vi "Calibrate Pneumotach.vi"(11 "Error In":errorcluster) -> (15 "Error Out":errorcluster)   [LabVIEW 2020]
uses:
  <vilib>/Analysis/baseanly.llb/Mean (DBL).vi
  <vilib>/measure/madcrms.llb/Basic Averaged DC-RMS for 1 Chan.vi
  <vilib>/gmath/NI_Gmath.lvlib
  <vilib>/Analysis/NI_AALBase.lvlib
  <vilib>/measure/NI_MAPro.lvlib
panel:
  in  "Remove Button":bool
  out "Flow Array":dbl[](array[numeric]) format="%_6g"
  out "Flow Calibration":cluster{"Y":dbl[], "Y":dbl[]}[](graph)
  out "Pressure Slope":dbl
  out "Pressure Intercept":dbl
  out "Pressure Voltage":dbl
  out "Flow Voltage":dbl
  in  "Flow Reference":dbl min=0.0 max=30.0 step=6.0
  out "Flow Intercept":dbl
  out "Flow Slope":dbl
  in  "Stop Button HS":bool
  in  "Add Button HS":bool
  out "Flow Curve":cluster{"Y":dbl[], "Y":dbl[]}[](graph)
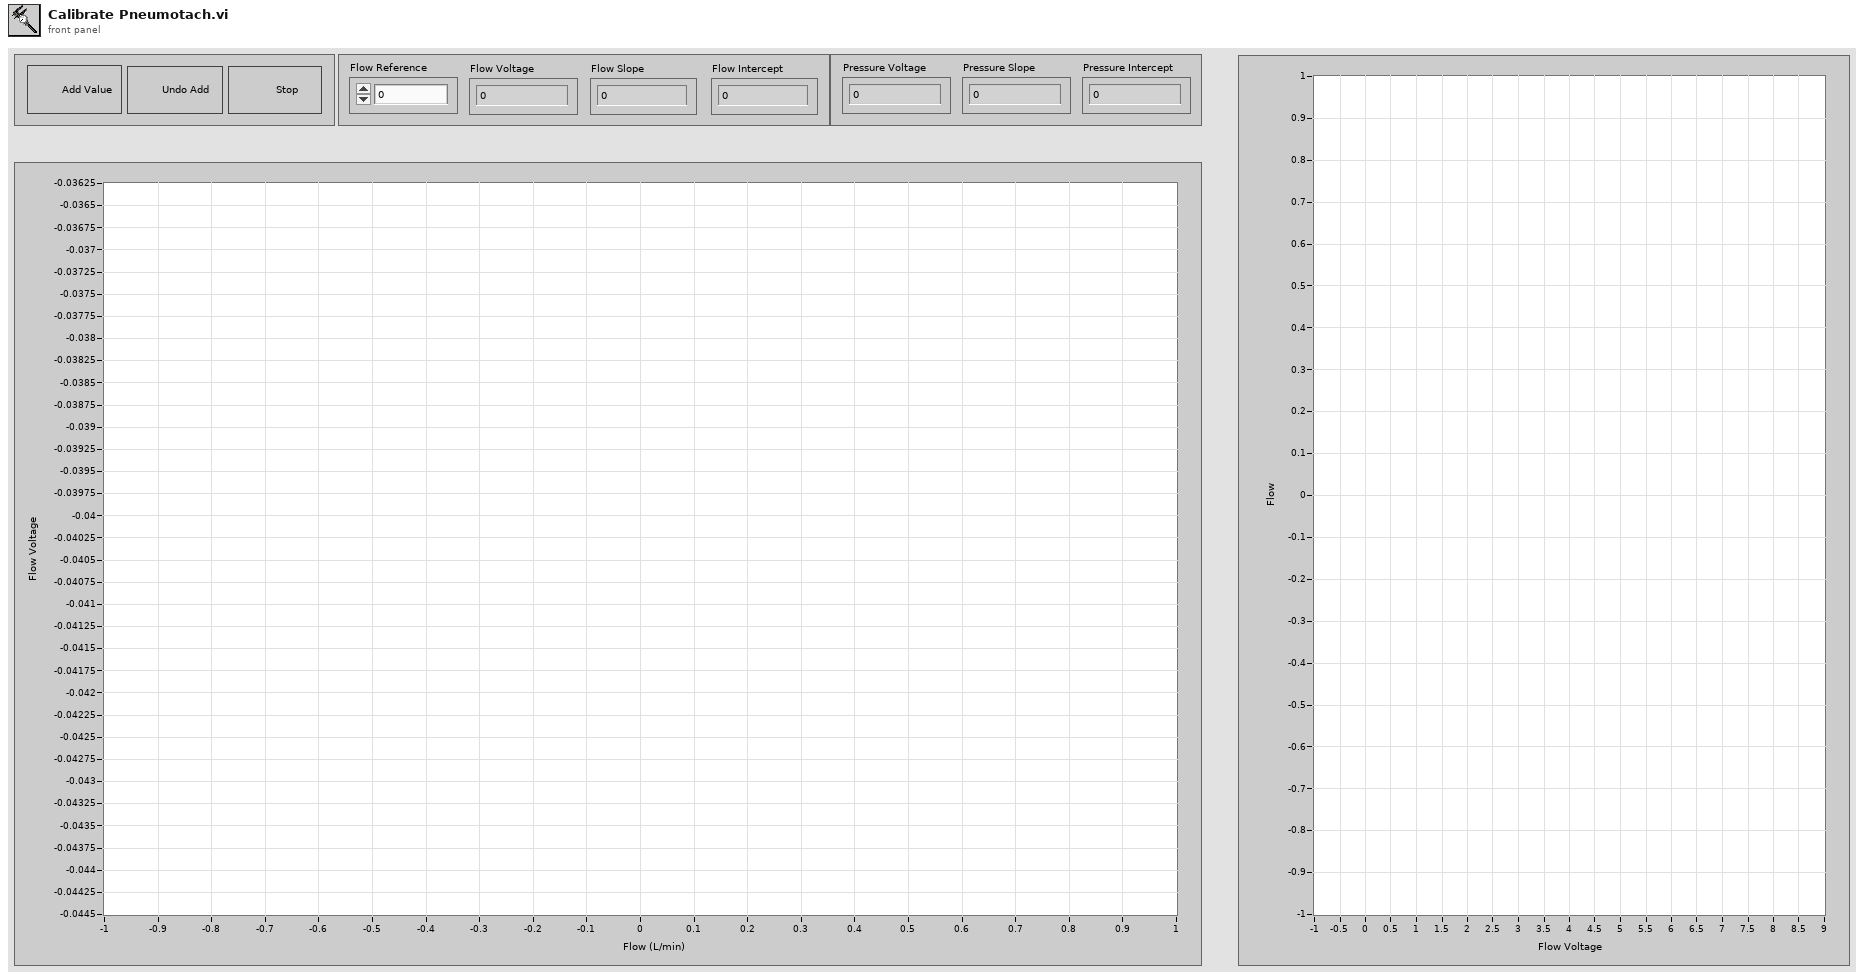
[diagram p1: front panel]
types:
  T1 = enum16{"open", "replace", "create", "open or create", "replace or create", "replace or create with confirmation"}
  T2 = enum8{"Enabled", "Disabled", "Disabled and Grayed Out"}
  T3 = cluster{"Volt (Flow)":dbl[], "Ref (Flow)":dbl[]}[]
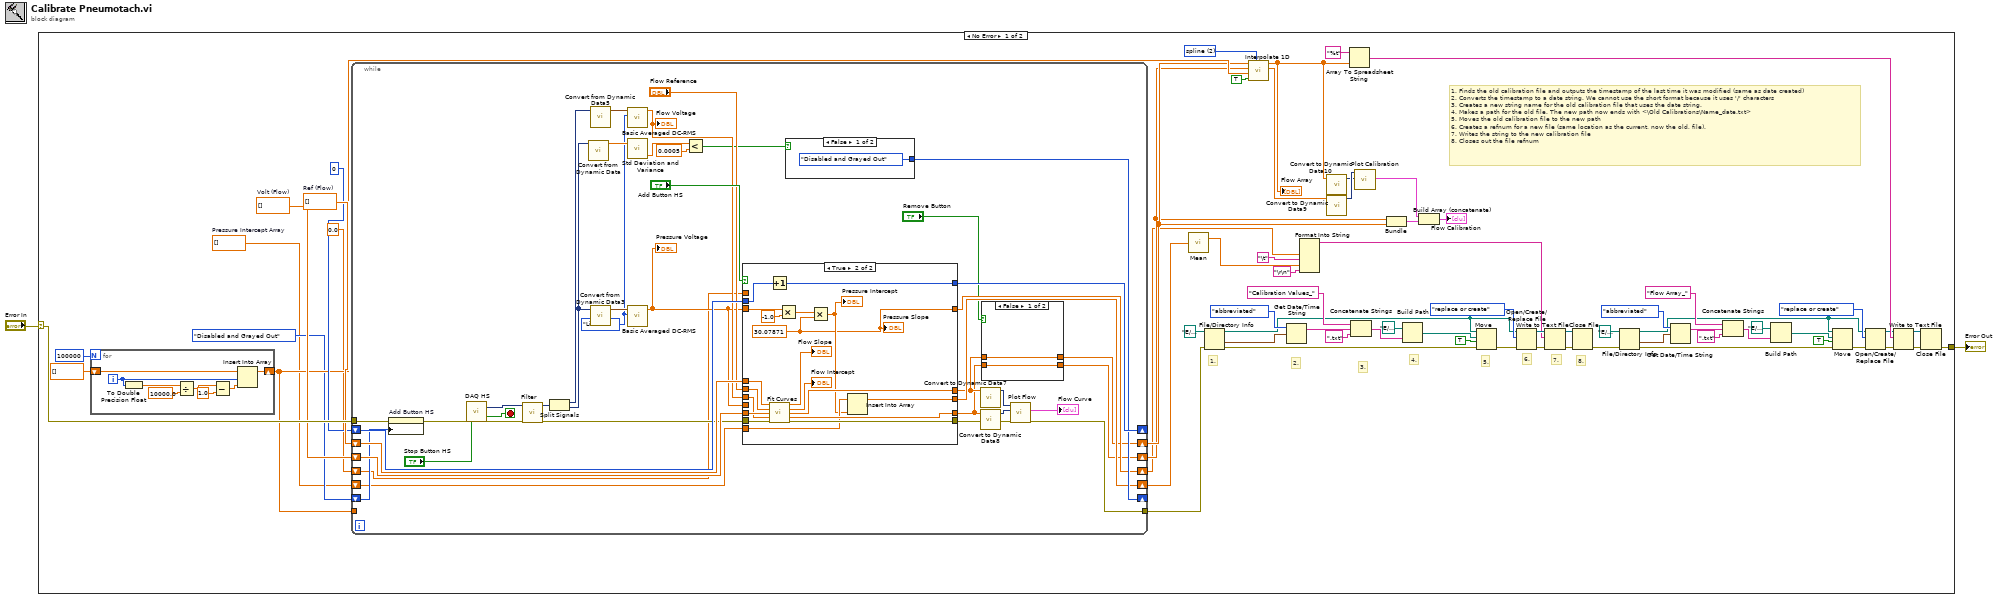
[diagram p0: block diagram]
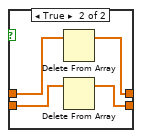
[diagram p2: hidden frame]
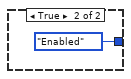
[diagram p3: hidden frame]
diagram:
  n1 = case shown="No Error" "Error In" {
    selector: "Error In" -> [w70 w153]
    tunnel: [w43 w153] -> w1
    frame No Error {
      w24 = dbl[] []  # Pressure Intercept Array
      w65 = 2 items=["nearest", "linear", "spline", "cubic Hermite", "Lagrange"] ("method")
      w68 = dbl[] []  # Ref (Flow)
      w69 = dbl[] []  # Volt (Flow)
      # "1. Finds the old calibration file and outputs the timestamp of the last time it was modified (same as date created)\n2. Converts the timestamp to a date string. We cannot use the short format because it uses '/' characters\n3. Creates a new string name for the old calibration file that uses the date string.\n4. Makes a path for the old file. The new path now ends with <\\Old Calibrations\\Name_date.txt>\n5. Moves the old calibration file to the new path\n6. Creates a refnum for a new file (same location as the current, now the old, file).\n7. Writes the string to the new calibration file\n8. Closes out the file refnum"
      # "8."
      # "7."
      # "6."
      # "5."
      # "4."
      # "3."
      # "2."
      # "1."
      n2 = for {
        N: 100000 ("dimension size") -> [_]
        shift-right: [w77] -> w59
        shift-left: dbl[] [] -> [w78]
        i -> [w74]
        n3 = To Double Precision Float(number=w74) -> (double precision float=w75:dbl)
        n4 = Divide(x=w75, y=10000.0) -> (x/y=w73:dbl)
        n5 = Subtract(x=w73, y=1.0) -> (x-y=w71:dbl)
        n6 = Insert Into Array(array=w78, index=w74, new element=w71) -> (w77:dbl[])
      }
      n7 = while {
        tunnel: w70 -> [w103]
        shift-right: [w79] -> w54
        shift-left: w69 -> [w106]
        shift-right: [w81] -> w55
        shift-left: w68 -> [w108]
        tunnel: [w111] -> w33
        shift-right: [w109] -> _
        shift-left: 0 -> [w110]
        tunnel: w59 -> [_]
        shift-right: [w100] -> _
        shift-left: T2."Disabled and Grayed Out" ("Disabled") -> [w101]
        shift-right: [w86] -> w23
        shift-left: w24 -> [w87]
        shift-right: [w84] -> w4
        shift-left: 0.0 -> [w85]
        stop <- w115 stop-if-true
        w92 = enum16{"Linear", "Exponential"}."Linear" ("averaging type")
        n8 = property on="Add Button HS" class="Bool"(error in=w103, "DisabledEnum"=w101) -> (error out=w102:errorcluster)  [unwired: 1 in, 1 out]
        n9 = call "DAQ HS"("error in"=w102, "stop (F)"="Stop Button HS") -> ("data"=w118:dynamicdata, "stopped"=w115:bool, "error out"=w119:errorcluster)  [unwired: 14 in, 1 out]
        n10 = call "Filter"("error in (no error)"=w119, "Signal"=w118) -> ("error out"=w93:errorcluster, "Filtered Signal"=w104:dynamicdata)  [unwired: 8 in]
        n11 = Split Signals(w104) -> (w89:dynamicdata, w95:dynamicdata)  [unwired: 2 in]
        n12 = call "Convert from Dynamic Data"("Dynamic Data Type"=w95) -> ("Array"=w98:dbl[])  [unwired: 3 in]
        n13 = call "Convert from Dynamic Data5"("Dynamic Data Type"=w89) -> ("Waveform"=w94:waveform(dbl))  [unwired: 3 in]
        n14 = call "Convert from Dynamic Data3"("Dynamic Data Type"=w95) -> ("Waveform"=w96:waveform(dbl))  [unwired: 3 in]
        n15 = call-poly <vilib>:"Basic Averaged DC-RMS.vi"("averaging type"=w92, "signal in"=w94) -> ("DC value"=w91:dbl)  [unwired: 6 in, 3 out]
        "Flow Voltage" <- w91
        n16 = call <vilib>:"Std Deviation and Variance.vi"("X"=w98) -> ("variance"=w97:dbl)  [unwired: 1 in, 2 out]
        n17 = call-poly <vilib>:"Basic Averaged DC-RMS.vi"("averaging type"=w92, "signal in"=w96) -> ("DC value"=w88:dbl)  [unwired: 6 in, 3 out]
        "Pressure Voltage" <- w88
        n18 = Less?(x=w97, y=0.0005) -> (x < y?=w90:bool)
        n19 = case shown="True" "Add Button HS" {
          tunnel: w93 -> [w133 w149]
          tunnel: [w133 w150] -> w114
          tunnel: w110 -> [w132 w152]
          tunnel: [w132 w151] -> w109
          tunnel: w108 -> [w131 w148]
          tunnel: "Flow Reference" -> [_ w147]
          tunnel: w106 -> [w130 w146]
          tunnel: w91 -> [_ w145]
          tunnel: [w131 w142] -> w82
          tunnel: [w130 w141] -> w80
          tunnel: w88 -> [_ _]
          tunnel: w88 -> [_ w136]
          tunnel: [w128 w134] -> w84
          tunnel: w87 -> [w129 w140]
          tunnel: [w129 w139] -> w86
          tunnel: w85 -> [w128 _]
          frame False {
          }
          frame True {
            w134 = 30.07871
            n20 = Increment(x=w152) -> (x+1=w151:i32)
            n21 = call "Fit Curves.vi"("Reference (Array)"=w148, "Reference (Value)"=w147, "Voltage (Array)"=w146, "Voltage (Value)"=w145, "Error In"=w149) -> ("Slope"=→"Flow Slope":dbl, "Intercept"=→"Flow Intercept":dbl, "Reference Out"=w142:dbl[], "Voltage Out"=w141:dbl[], "Error Out"=w150:errorcluster)  [unwired: 6 in]
            n22 = Multiply(x=w136, y=-1.0) -> (x*y=w135:dbl)
            n23 = Multiply(x=w135, y=w134) -> (x*y=w137:dbl)
            "Pressure Intercept" <- w137
            n24 = Insert Into Array(array=w140, new element=w137) -> (w139:dbl[])  [unwired: 1 in]
            "Pressure Slope" <- w134
          }
        }
        n25 = case shown="False" w90 {
          tunnel: [T2."Disabled and Grayed Out" ("Disabled") T2."Enabled" ("Disabled")] -> w100
          frame False {
          }
          frame True {
          }
        }
        n26 = call "Convert to Dynamic Data7"("Array"=w82) -> ("Dynamic Data Type"=w112:dynamicdata)  [unwired: 3 in]
        n27 = call "Convert to Dynamic Data8"("Array"=w80) -> ("Dynamic Data Type"=w113:dynamicdata)  [unwired: 3 in]
        n28 = case shown="False" "Remove Button" {
          tunnel: w82 -> [w121 w125]
          tunnel: [w121 w124] -> w81
          tunnel: w80 -> [w120 w123]
          tunnel: [w120 w122] -> w79
          frame False {
          }
          frame True {
            n29 = Delete From Array(array=w125) -> (array with subset deleted=w124:dbl[])  [unwired: 2 in, 1 out]
            n30 = Delete From Array(array=w123) -> (array with subset deleted=w122:dbl[])  [unwired: 2 in, 1 out]
          }
        }
        n31 = call "Plot Flow"("error in (no error)"=w114, "Y Input"=w113, "X Input"=w112) -> ("error out"=w111:errorcluster, "XY Graph"=→"Flow Curve":cluster{"Y":dbl[], "Y":dbl[]}[])  [unwired: 7 in]
      }
      n32 = call-poly <vilib>:"Mean.vi"("X"=w23) -> ("mean"=w3:dbl)  [unwired: 1 out]
      n33 = File/Directory Info(path=path "E:/Program Files/Master Aero Program/Calibration .txt files/Calibration Values.txt" ("file path (use dialog)"), error in=w33) -> (path out=w26:path, last mod=w30:timestamp, error out=w34:errorcluster)  [unwired: 4 out]
      n34 = call <vilib>:"Interpolate 1D.vi"("method"=w65, "X is monotonic"=TRUE, "xi"=w59, "X"=w54, "Y"=w55) -> ("xi used"=w57:dbl[], "yi"=w46:dbl[])  [unwired: 4 in, 1 out]
      "Flow Array" <- w46
      n35 = Get Date/Time String(date format (0)=enum16{"short", "long", "abbreviated"}."abbreviated", seconds (now)=w30) -> (date string=w29:string)  [unwired: 1 in, 1 out]
      n36 = Format Into String(w4, "\t", w3, "\r\n") -> (resulting string=w49:string)  [unwired: 3 in, 1 out]
      n37 = call "Convert to Dynamic Data10"("Array"=w46) -> ("Dynamic Data Type"=w63:dynamicdata)  [unwired: 3 in]
      n38 = call "Convert to Dynamic Data9"("Array"=w57) -> ("Dynamic Data Type"=w64:dynamicdata)  [unwired: 3 in]
      n39 = Array To Spreadsheet String(array=w46, 3:"%t" ("format string")) -> (spreadsheet string=w41:string)  [unwired: 1 in]
      n40 = Concatenate Strings("Calibration Values_" ("string"), w29, ".txt" ("string")) -> (w36:string)
      n41 = call "Plot Calibration"("Y Input"=w63, "X Input"=w64) -> ("XY Graph"=w62:cluster{"Y":dbl[], "Y":dbl[]}[])  [unwired: 8 in, 1 out]
      n42 = Bundle("Volt (Flow)"=w54, "Ref (Flow)"=w55) -> (w61:cluster{"Volt (Flow)":dbl[], "Ref (Flow)":dbl[]})  [unwired: 1 in]
      n43 = Build Path(base path=path "E:/Program Files/Master Aero Program/Calibration .txt files/Old Calibrations" ("target path (use dialog)"), name or relative path=w36) -> (appended path=w39:path)
      n44 = Build Array (concatenate)(w62, w61) -> (→"Flow Calibration":T3)
      n45 = Move(source path=w26, error in=w34, 9:TRUE ("overwrite (F)"), 10:w39) -> (error out=w40:errorcluster)  [unwired: 1 in, 2 out]
      n46 = Open/Create/Replace File(file path (use dialog)=w26, error in=w40, operation (0:open)=T1."replace or create") -> (refnum out=w51:refnum<file>, error out=w35:errorcluster)  [unwired: 3 in, 1 out]
      n47 = Write to Text File(file (use dialog)=w51, text=w49, error in=w35) -> (refnum out=w50:refnum<file>, error out=w52:errorcluster)  [unwired: 1 in, 1 out]
      n48 = Close File(refnum=w50, error in=w52) -> (error out=w28:errorcluster)  [unwired: 1 out]
      n49 = File/Directory Info(path=path "E:/Program Files/Master Aero Program/Calibration .txt files/Flow Array.txt" ("file path (use dialog)"), error in=w28) -> (path out=w6:path, last mod=w8:timestamp, error out=w15:errorcluster)  [unwired: 4 out]
      n50 = Get Date/Time String(date format (0)=enum16{"short", "long", "abbreviated"}."abbreviated", seconds (now)=w8) -> (date string=w7:string)  [unwired: 1 in, 1 out]
      n51 = Concatenate Strings("Flow Array_" ("string"), w7, ".txt" ("string")) -> (w12:string)
      n52 = Build Path(base path=path "E:/Program Files/Master Aero Program/Calibration .txt files/Old Calibrations" ("target path (use dialog)"), name or relative path=w12) -> (appended path=w16:path)
      n53 = Move(source path=w6, error in=w15, 9:TRUE ("overwrite (F)"), 10:w16) -> (error out=w17:errorcluster)  [unwired: 1 in, 2 out]
      n54 = Open/Create/Replace File(file path (use dialog)=w6, error in=w17, operation (0:open)=T1."replace or create") -> (refnum out=w20:refnum<file>, error out=w19:errorcluster)  [unwired: 3 in, 1 out]
      n55 = Write to Text File(file (use dialog)=w20, text=w41, error in=w19) -> (refnum out=w21:refnum<file>, error out=w18:errorcluster)  [unwired: 1 in, 1 out]
      n56 = Close File(refnum=w21, error in=w18) -> (error out=w43:errorcluster)  [unwired: 1 out]
    }
    frame Error {
    }
  }
  "Error Out" <- w1
